vi "回文数质数算法1改1.vi"(3 "上限":dbl) -> (0 "回文质数数量":dbl, 1 "回文质数":dbl[](array[numeric]))   [LabVIEW 2017]
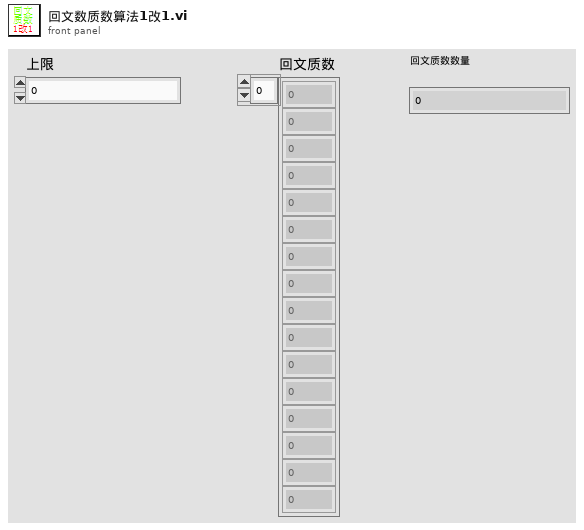
[diagram p1: front panel]
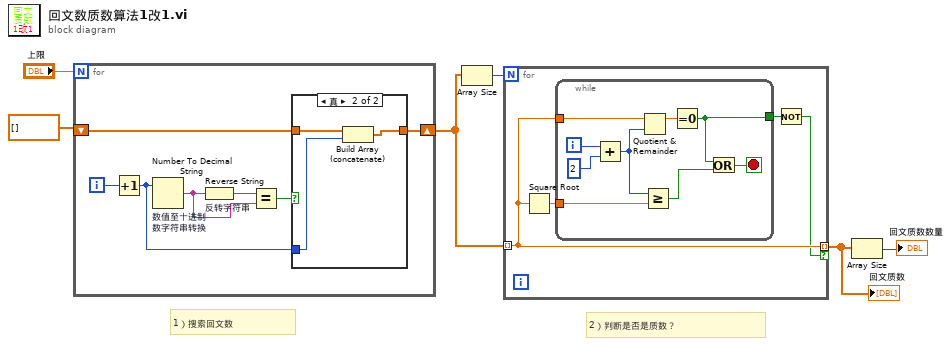
[diagram p0: block diagram]
diagram:
  # "2）判断是否是质数？"
  # "1）搜索回文数"
  n1 = for {
    N: "上限" -> [_]
    shift-right: [w11] -> w4
    shift-left: dbl[] [] -> [w12]
    i -> [w13]
    n2 = Increment(x=w13) -> (x+1=w9:i32)
    n3 = Number To Decimal String "数值至十进制\n数字符串转换"(number=w9) -> (decimal integer string=w7:string)  [unwired: 1 in]
    n4 = Reverse String "反转字符串"(1:w7) -> (0:w8:string)
    n5 = Equal?(x=w8, y=w7) -> (x = y?=w10:bool)
    n6 = case shown="真" w10 {
      tunnel: w12 -> [w14 w17]
      tunnel: [w14 w16] -> w11
      tunnel: w9 -> [_ w15]
      frame False {
      }
      frame True {
        n7 = Build Array (concatenate)(w17, w15) -> (w16:dbl[])
      }
    }
  }
  n8 = Array Size(array=w4) -> (size(s)=w6:i32)
  n9 = for {
    N: w6 -> [_]
    tunnel: w4 -> [w19] mode=indexing
    tunnel: [w19] -> w1 mode=indexing if=w18
    n10 = Square Root(x=w19) -> (sqrt(x)=w21:dbl)
    n11 = while {
      tunnel: w21 -> [w26]
      tunnel: [w22] -> w20
      tunnel: w19 -> [w23]
      i -> [w29]
      stop <- w30 stop-if-true
      n12 = Add(x=w29, y=2) -> (x+y=w24:i32)
      n13 = Quotient & Remainder(x=w23, y=w24) -> (x-y*floor(x/y)=w27:dbl)  [unwired: 1 out]
      n14 = Greater Or Equal?(x=w24, y=w26) -> (x >= y?=w25:bool)
      n15 = Equal To 0?(x=w27) -> (x = 0?=w22:bool)
      n16 = Or(x=w22, y=w25) -> (x .or. y?=w30:bool)
    }
    n17 = Not(x=w20) -> (.not. x?=w18:bool)
  }
  "回文质数" <- w1
  n18 = Array Size(array=w1) -> (size(s)=→"回文质数数量":i32)
